vi "BM0211 Image property read write.vi"(9 "Read write":enum16{"write", "Read"}(ring)=enum."Read", 11 "IN":T1(array[cluster])) -> (0 "error out":errorcluster, 3 "Out":T1(array[cluster]))   [LabVIEW 2015]
uses:
  Galobal variable_TI.vi
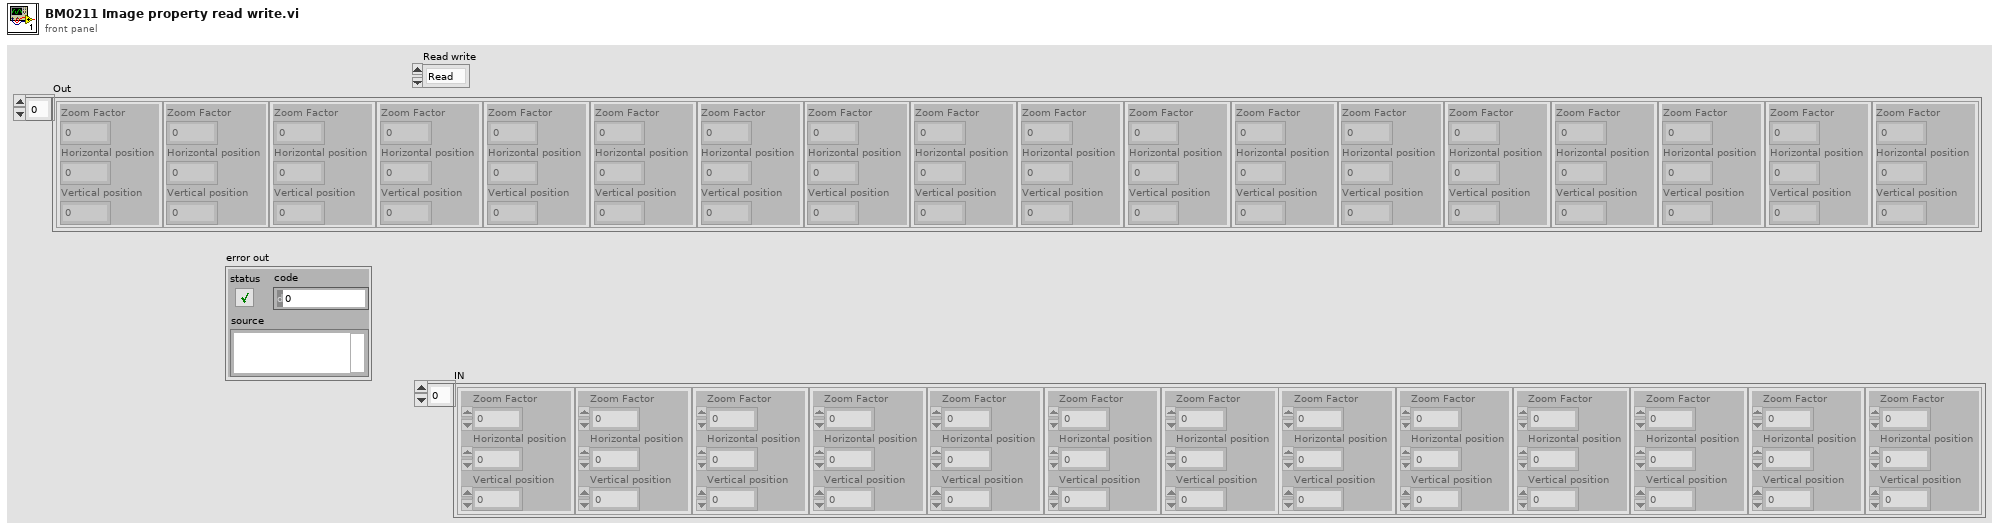
[diagram p1: front panel]
types:
  T1 = cluster{"Zoom Factor":sgl, "Horizontal position":sgl, "Vertical position":sgl}[]
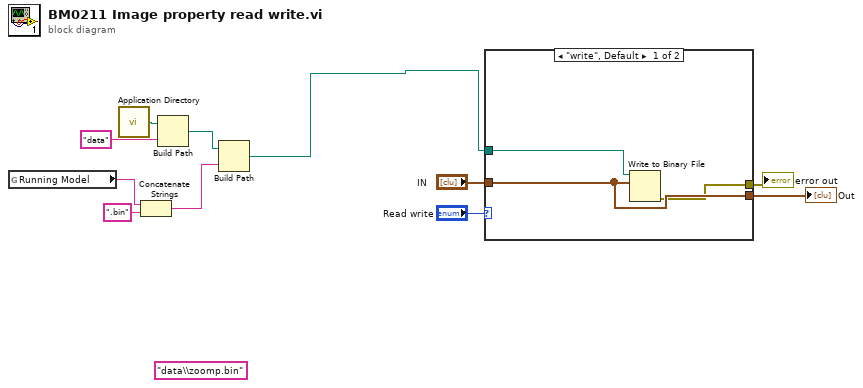
[diagram p0: block diagram]
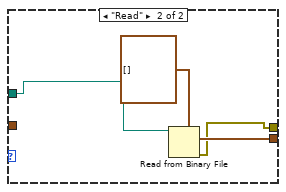
[diagram p2: hidden frame]
diagram:
  (unwired) "data\\zoomp.bin" ("name or relative path")
  n1 = global read "Galobal variable_TI.vi" "Running Model"() -> (w4:string)
  n2 = call <vilib>:"Application Directory.vi"() -> ("Application Directory"=w7:path)
  n3 = Concatenate Strings(w4, ".bin" ("string")) -> (w2:string)
  n4 = Build Path(base path=w7, name or relative path="data") -> (appended path=w5:path)
  n5 = Build Path(base path=w5, name or relative path=w2) -> (appended path=w1:path)
  n6 = case shown="\"write\", Default" "Read write" {
    tunnel: "IN" -> [w13 _]
    tunnel: w1 -> [w14 w18]
    tunnel: [w13 w16] -> w9
    tunnel: [w12 w15] -> w8
    frame "write", Default {
      n7 = Write to Binary File(file (use dialog)=w14, data=w13) -> (error out=w12:errorcluster)  [unwired: 4 in, 2 out]
    }
    frame "Read" {
      n8 = Read from Binary File(5:T1 [] ("Array"), 11:w18) -> (0:w15:errorcluster, 2:w16:T1)  [unwired: 4 in, 2 out]
    }
  }
  "Out" <- w9
  "error out" <- w8
